vi "Illumination Tests_3.vi"(0 "Test Number":i32, 5 "FileName":path=path "c:/$safe$.bmp", 7 "Pixel Offset":i32, 9 "Pixel Average":i32) -> (1 "Hor Max":sgl format="%.2g", 2 "Vert Max":sgl format="%#.2g", 3 "Gray Level Intensity":T2 {"Standard  Deviation" format="%.2f"; "Mean Intensity" format="%.2f"; "Maximum Intensity" format="%.2f"; "Minimum Intensity" format="%.2f"}, 4 "Mean Intensity":sgl, 6 "Horz Ratio":sgl format="%#.2g", 10 "Vert Ratio":sgl format="%#.2g", 12 "Horz Min":sgl format="%.2g", 14 "Vert Min":sgl format="%#.2g", 15 "error out":errorcluster)   [LabVIEW 2014]
uses:
  <vilib>/vision/NI_Vision_Development_Module.lvlib
panel:
  out "X Resolution Center":i32
  out "Y Resolution Center":i32
  out "Y Resolution":i32
  out "X Resolution":i32
  out "Image":T1(plugin-control)
  out "Vertical Averages":sgl[](array[numeric]) format="%#.2g"
  out "Horizontal Averages":sgl[](array[numeric]) format="%#.2g"
  in  "error in (no error)":errorcluster
  # "0 = Center Illumination Brightness\n1 = Uniformity\n2 = Spot Color Test"
  # "UNIFORMITY"
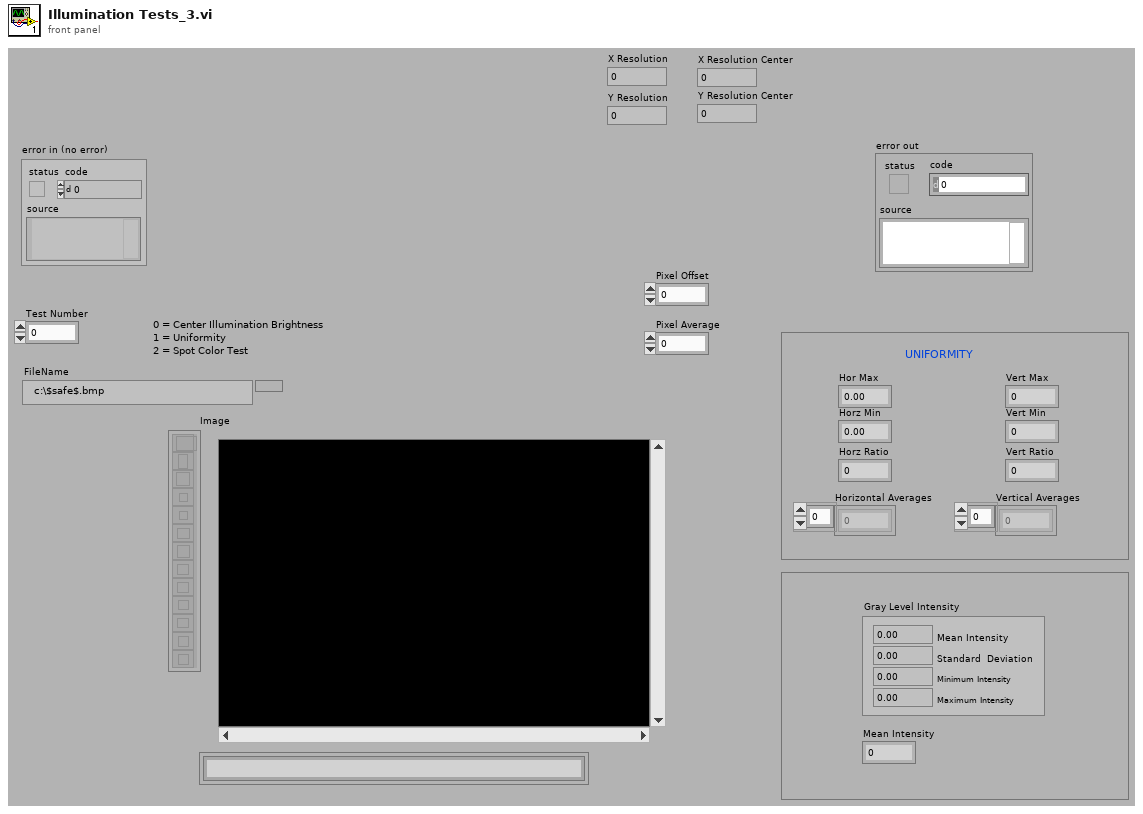
[diagram p1: front panel]
types:
  T1 = typedef "IMAQ Image.ctl" = refnum<image>
  T2 = cluster{"Mean Intensity":sgl, "Standard  Deviation":sgl, "Minimum Intensity":sgl, "Maximum Intensity":sgl}
  T3 = typedef "IMAQ Rectangle" = cluster{"Left":i32, "Top":i32, "Right":i32, "Bottom":i32, "Rotation":dbl}
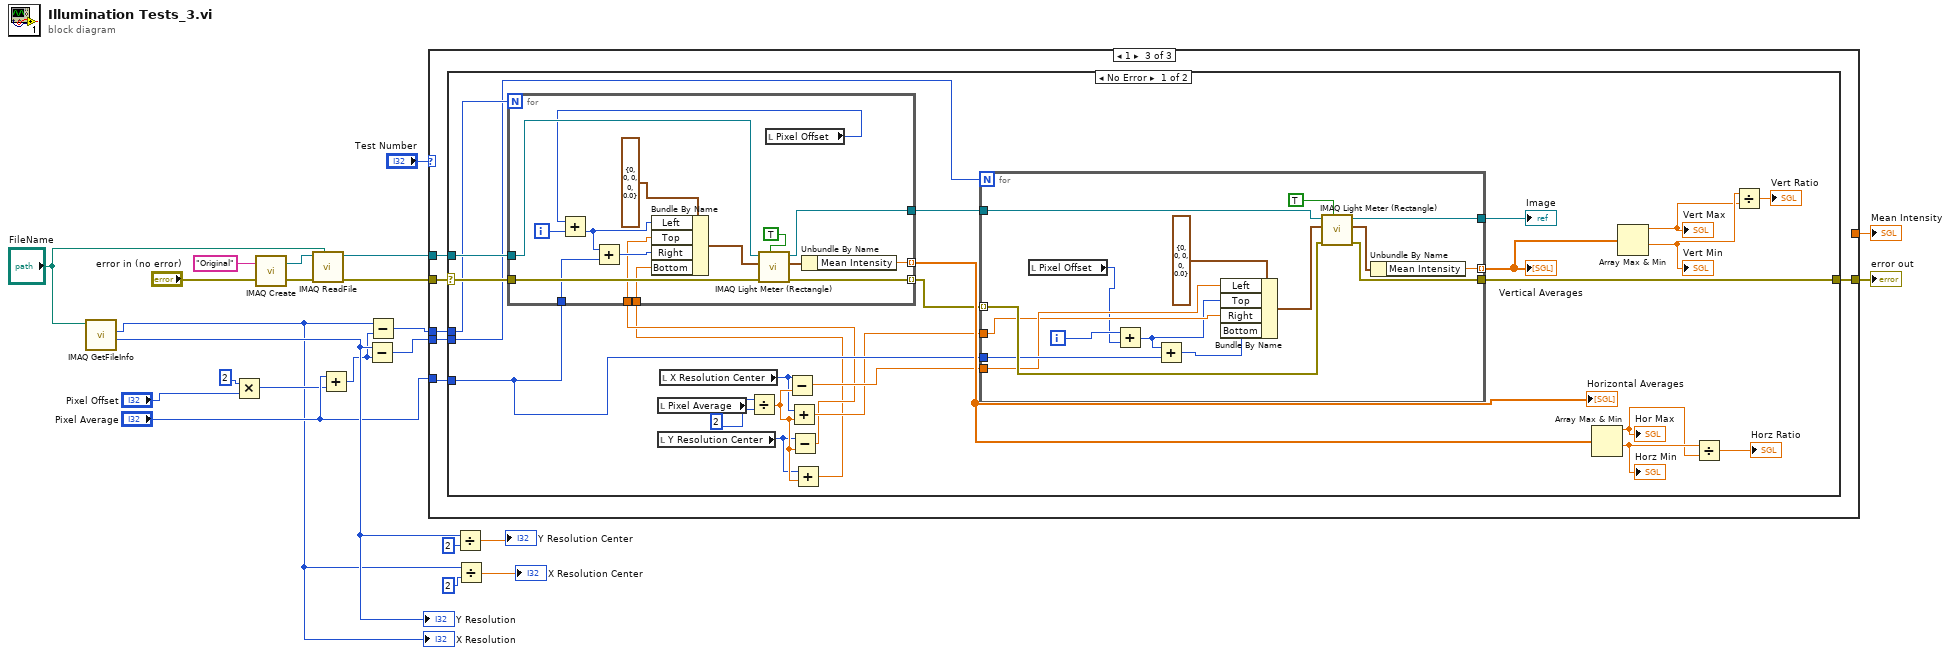
[diagram p0: block diagram]
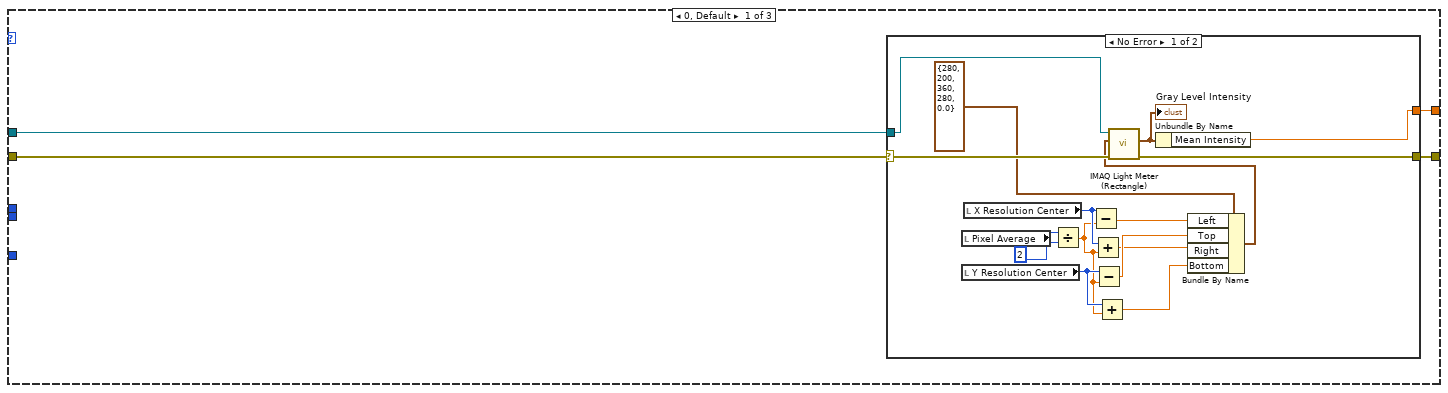
[diagram p2: hidden frame]
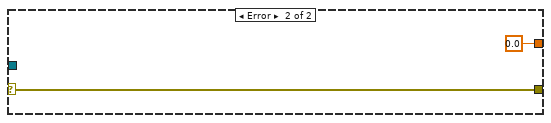
[diagram p3: hidden frame]
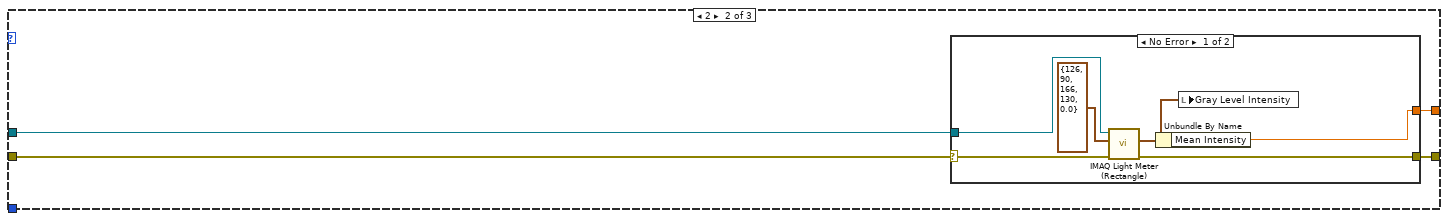
[diagram p4: hidden frame]
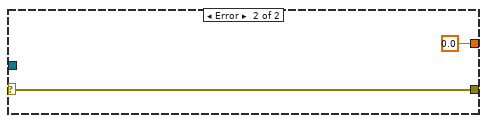
[diagram p5: hidden frame]
diagram:
  n1 = call "IMAQ GetFileInfo"("File Path"="FileName") -> ("Y Resolution"=w13:i32, "X Resolution"=w1:i32)  [unwired: 4 in, 5 out]
  "X Resolution" <- w1
  "Y Resolution" <- w13
  n2 = Multiply(x=2, y="Pixel Offset") -> (x*y=w5:i32)
  n3 = call "IMAQ Create"("Image Name"="Original", "error in (no error)"="error in (no error)") -> ("New Image"=w22:T1, "error out"=w19:errorcluster)  [unwired: 3 in]
  n4 = call "IMAQ ReadFile"("File Path"="FileName", "error in (no error)"=w19, "Image"=w22) -> ("error out"=w18:errorcluster, "Image Out"=w21:T1)  [unwired: 4 in, 3 out]
  n5 = Add(x="Pixel Average", y=w5) -> (x+y=w2:i32)
  n6 = Subtract(x=w13, y=w2) -> (x-y=w14:i32)
  n7 = Subtract(x=w1, y=w2) -> (x-y=w3:i32)
  n8 = case shown="1" "Test Number" {
    tunnel: w21 -> [w27 w49 w61]
    tunnel: w18 -> [w26 w48 w63]
    tunnel: [w25 w47 _] -> w17
    tunnel: [w24 w46 w62] -> w16
    tunnel: w3 -> [_ _ w60]
    tunnel: w14 -> [_ _ w59]
    tunnel: "Pixel Average" -> [_ _ w58]
    frame 0, Default {
      n9 = case shown="No Error" w26 {
        selector: w26 -> [w39 w44]
        tunnel: w27 -> [w43 _]
        tunnel: [w41 sgl 0.0 ("Mean Intensity")] -> w25
        tunnel: [w40 w44] -> w24
        frame No Error {
          n10 = local read "Pixel Average"() -> (w33:i32)
          n11 = local read "Y Resolution Center"() -> (w34:i32)
          n12 = local read "X Resolution Center"() -> (w35:i32)
          n13 = Divide(x=w33, y=2) -> (x/y=w29:dbl)
          n14 = Subtract(x=w35, y=w29) -> (x-y=w36:dbl)
          n15 = Add(x=w35, y=w29) -> (x+y=w30:dbl)
          n16 = Subtract(x=w34, y=w29) -> (x-y=w32:dbl)
          n17 = Add(x=w34, y=w29) -> (x+y=w31:dbl)
          n18 = Bundle By Name(cluster=T3 {"Left"=280, "Top"=200, "Right"=360, "Bottom"=280, "Rotation"=0.0} ("Rectangle"), "Left"=w36, "Top"=w32, "Right"=w30, "Bottom"=w31) -> (w38:T3)
          n19 = call "IMAQ Light Meter (Rectangle)"("error in (no error)"=w39, "Rectangle"=w38, "Image"=w43) -> ("error out"=w40:errorcluster, "Gray Level Intensities"=w42:T2)  [unwired: 4 in, 3 out]
          "Gray Level Intensity" <- w42
          n20 = Unbundle By Name(w42) -> ("Mean Intensity"=w41:sgl)
        }
        frame Error {
        }
      }
    }
    frame 2 {
      n21 = case shown="No Error" w48 {
        selector: w48 -> [w51 w56]
        tunnel: w49 -> [w54 _]
        tunnel: [w53 sgl 0.0 ("Mean Intensity")] -> w47
        tunnel: [w52 w56] -> w46
        frame No Error {
          n22 = call "IMAQ Light Meter (Rectangle)"("error in (no error)"=w51, "Rectangle"=T3 {"Left"=126, "Top"=90, "Right"=166, "Bottom"=130, "Rotation"=0.0}, "Image"=w54) -> ("error out"=w52:errorcluster, "Gray Level Intensities"=w50:T2)  [unwired: 4 in, 3 out]
          n23 = Unbundle By Name(w50) -> ("Mean Intensity"=w53:sgl)
          n24 = local write "Gray Level Intensity"(w50) -> ()
        }
        frame Error {
        }
      }
    }
    frame 1 {
      n25 = case shown="No Error" w63 {
        selector: w63 -> [w80 w122]
        tunnel: [w79 w122] -> w62
        tunnel: w61 -> [w76 _]
        tunnel: w60 -> [w75 _]
        tunnel: w59 -> [w74 _]
        tunnel: w58 -> [w73 _]
        frame No Error {
          n26 = local read "Pixel Average"() -> (w70:i32)
          n27 = local read "Y Resolution Center"() -> (w69:i32)
          n28 = local read "X Resolution Center"() -> (w68:i32)
          n29 = Divide(x=w70, y=2) -> (x/y=w71:dbl)
          n30 = Subtract(x=w68, y=w71) -> (x-y=w67:dbl)
          n31 = Add(x=w68, y=w71) -> (x+y=w66:dbl)
          n32 = Subtract(x=w69, y=w71) -> (x-y=w65:dbl)
          n33 = Add(x=w69, y=w71) -> (x+y=w64:dbl)
          n34 = for {
            N: w75 -> [_]
            tunnel: [w116] -> w89 mode=indexing
            tunnel: w76 -> [w114]
            tunnel: [w113] -> w81 mode=indexing
            tunnel: w80 -> [w112]
            tunnel: [w111] -> w78
            tunnel: w73 -> [w110]
            tunnel: w65 -> [w109]
            tunnel: w64 -> [w108]
            i -> [w120]
            n35 = local read "Pixel Offset"() -> (w106:i32)
            n36 = Add(x=w106, y=w120) -> (x+y=w107:i32)
            n37 = Add(x=w107, y=w110) -> (x+y=w119:i32)
            n38 = Bundle By Name(cluster=T3 {"Left"=0, "Top"=0, "Right"=0, "Bottom"=0, "Rotation"=0.0} ("Rectangle"), "Left"=w107, "Top"=w109, "Right"=w119, "Bottom"=w108) -> (w118:T3)
            n39 = call "IMAQ Light Meter (Rectangle)"("Show Search Area"=TRUE, "error in (no error)"=w112, "Rectangle"=w118, "Image"=w114) -> ("error out"=w113:errorcluster, "Gray Level Intensities"=w117:T2, "Image Out"=w111:T1)  [unwired: 3 in, 2 out]
            n40 = Unbundle By Name(w117) -> ("Mean Intensity"=w116:sgl)
          }
          "Horizontal Averages" <- w89
          n41 = for {
            N: w74 -> [_]
            tunnel: [w102] -> w88 mode=indexing
            tunnel: [w101] -> w79
            tunnel: w81 -> [w97] mode=indexing
            tunnel: w78 -> [w96]
            tunnel: [w95] -> w77
            tunnel: w73 -> [w94]
            tunnel: w67 -> [w93]
            tunnel: w66 -> [w92]
            i -> [w99]
            n42 = local read "Pixel Offset"() -> (w90:i32)
            n43 = Add(x=w99, y=w90) -> (x+y=w91:i32)
            n44 = Add(x=w91, y=w94) -> (x+y=w98:i32)
            n45 = Bundle By Name(cluster=T3 {"Left"=0, "Top"=0, "Right"=0, "Bottom"=0, "Rotation"=0.0} ("Rectangle"), "Left"=w93, "Top"=w91, "Right"=w92, "Bottom"=w98) -> (w104:T3)
            n46 = call "IMAQ Light Meter (Rectangle)"("Show Search Area"=TRUE, "error in (no error)"=w97, "Rectangle"=w104, "Image"=w96) -> ("error out"=w101:errorcluster, "Gray Level Intensities"=w103:T2, "Image Out"=w95:T1)  [unwired: 3 in, 2 out]
            n47 = Unbundle By Name(w103) -> ("Mean Intensity"=w102:sgl)
          }
          "Vertical Averages" <- w88
          "Image" <- w77
          n48 = Array Max & Min(array=w89) -> (max value=w84:sgl, min value=w85:sgl)  [unwired: 2 out]
          "Hor Max" <- w84
          "Horz Min" <- w85
          n49 = Array Max & Min(array=w88) -> (max value=w86:sgl, min value=w87:sgl)  [unwired: 2 out]
          "Vert Max" <- w86
          "Vert Min" <- w87
          n50 = Divide(x=w85, y=w84) -> (x/y=→"Horz Ratio":sgl)
          n51 = Divide(x=w87, y=w86) -> (x/y=→"Vert Ratio":sgl)
        }
        frame Error {
        }
      }
    }
  }
  "Mean Intensity" <- w17
  "error out" <- w16
  n52 = Divide(x=w13, y=2) -> (x/y=→"Y Resolution Center":dbl)
  n53 = Divide(x=w1, y=2) -> (x/y=→"X Resolution Center":dbl)
